vi "ImageNoiseBlock1Image.vi"(3 "BERHP":sgl) -> (9 "High-Power Image":T1(plugin-control))   [LabVIEW 2022 SP3]
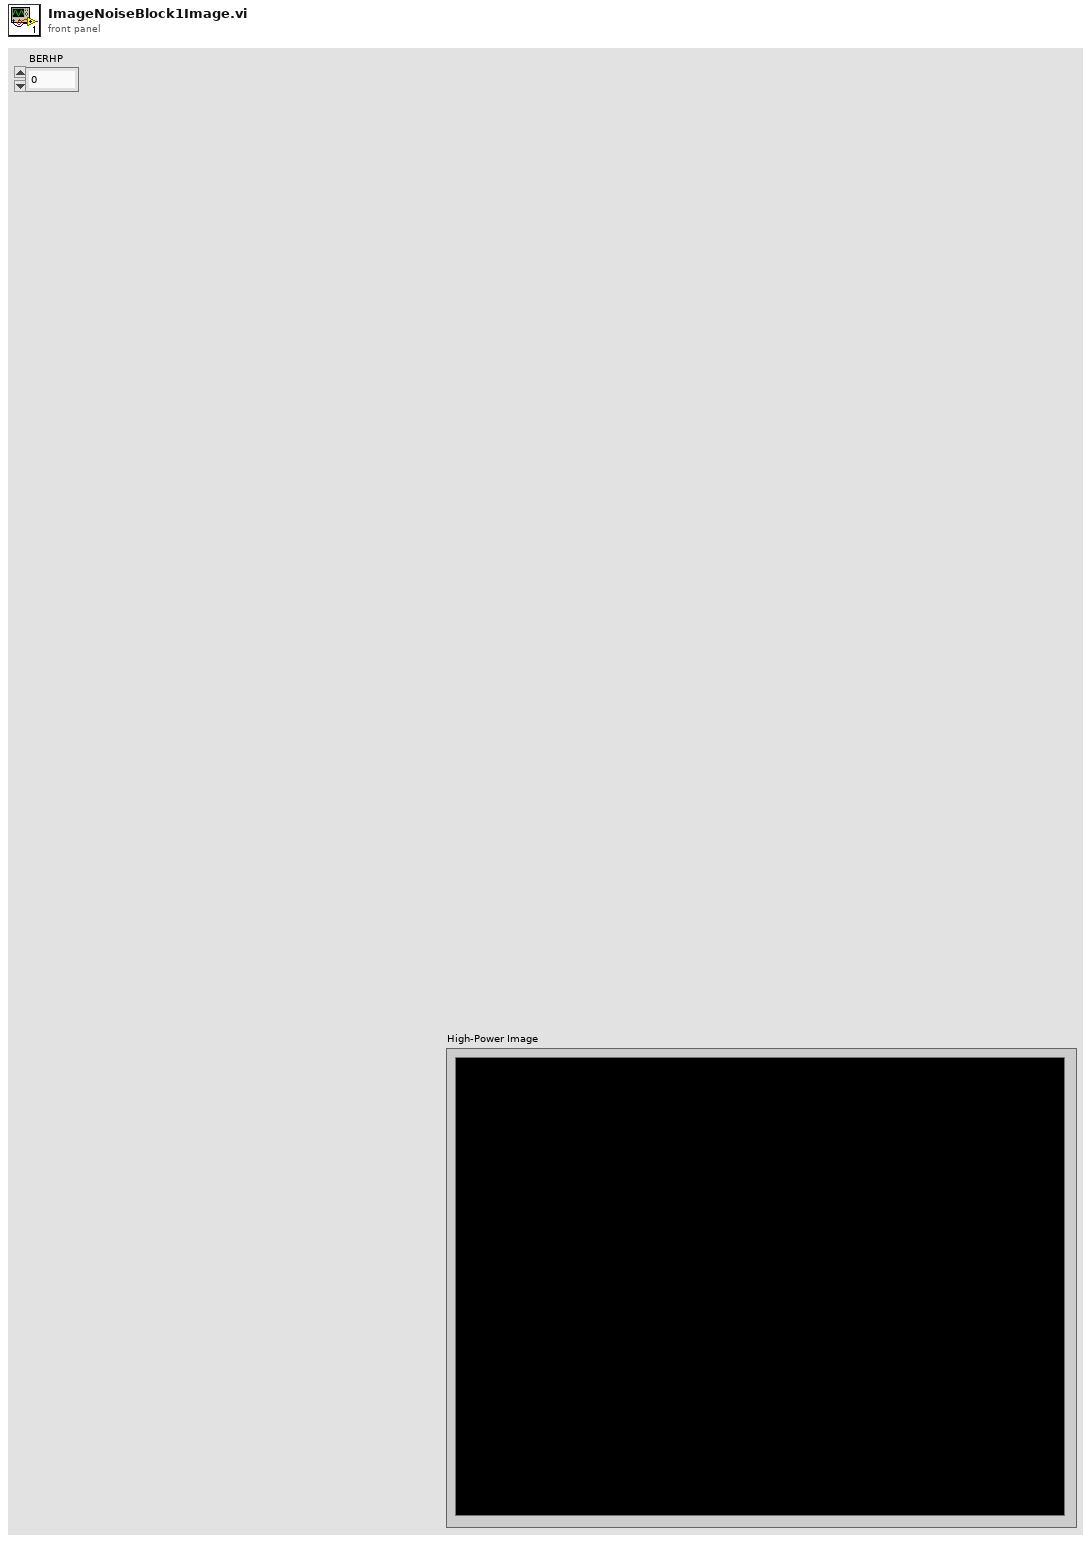
[diagram p1: front panel]
types:
  T1 = typedef "IMAQ Image.ctl" = refnum<image>
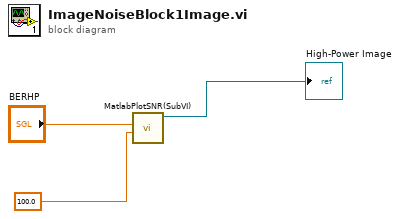
[diagram p0: block diagram]
diagram:
  n1 = call "MatlabPlotSNR(SubVI).vi"("BERLP"=100.0, "BERHP"="BERHP") -> ("Refnum out HP"=→"High-Power Image":T1)  [unwired: 8 in, 1 out]
